vi "RealTimeConversions-CSV.vi"() -> ()   [LabVIEW 2019]
uses:
  <vilib>/userDefined/High Color/IMAQdx.ctl
  <vilib>/vision/driver/NI_Vision_Acquisition_Software.lvlib
  RGB_To_Gray DLL Project/Project RGBToGray VI/RGBToGray.dll
  Gray_To_RGB DLL Project/Gray_to_RGB.dll
panel:
  out "RGB Frame":T1(plugin-control)
  out "GrayScale Frame":T1(plugin-control)
  out "Array":dbl[](array[numeric])
  in  "CSV File Path":path
  out "Elapsed time RGB in sec":dbl
  in  "stop":bool
  out "Camera Frame":T1(plugin-control)
  in  "Available Colormaps":T2
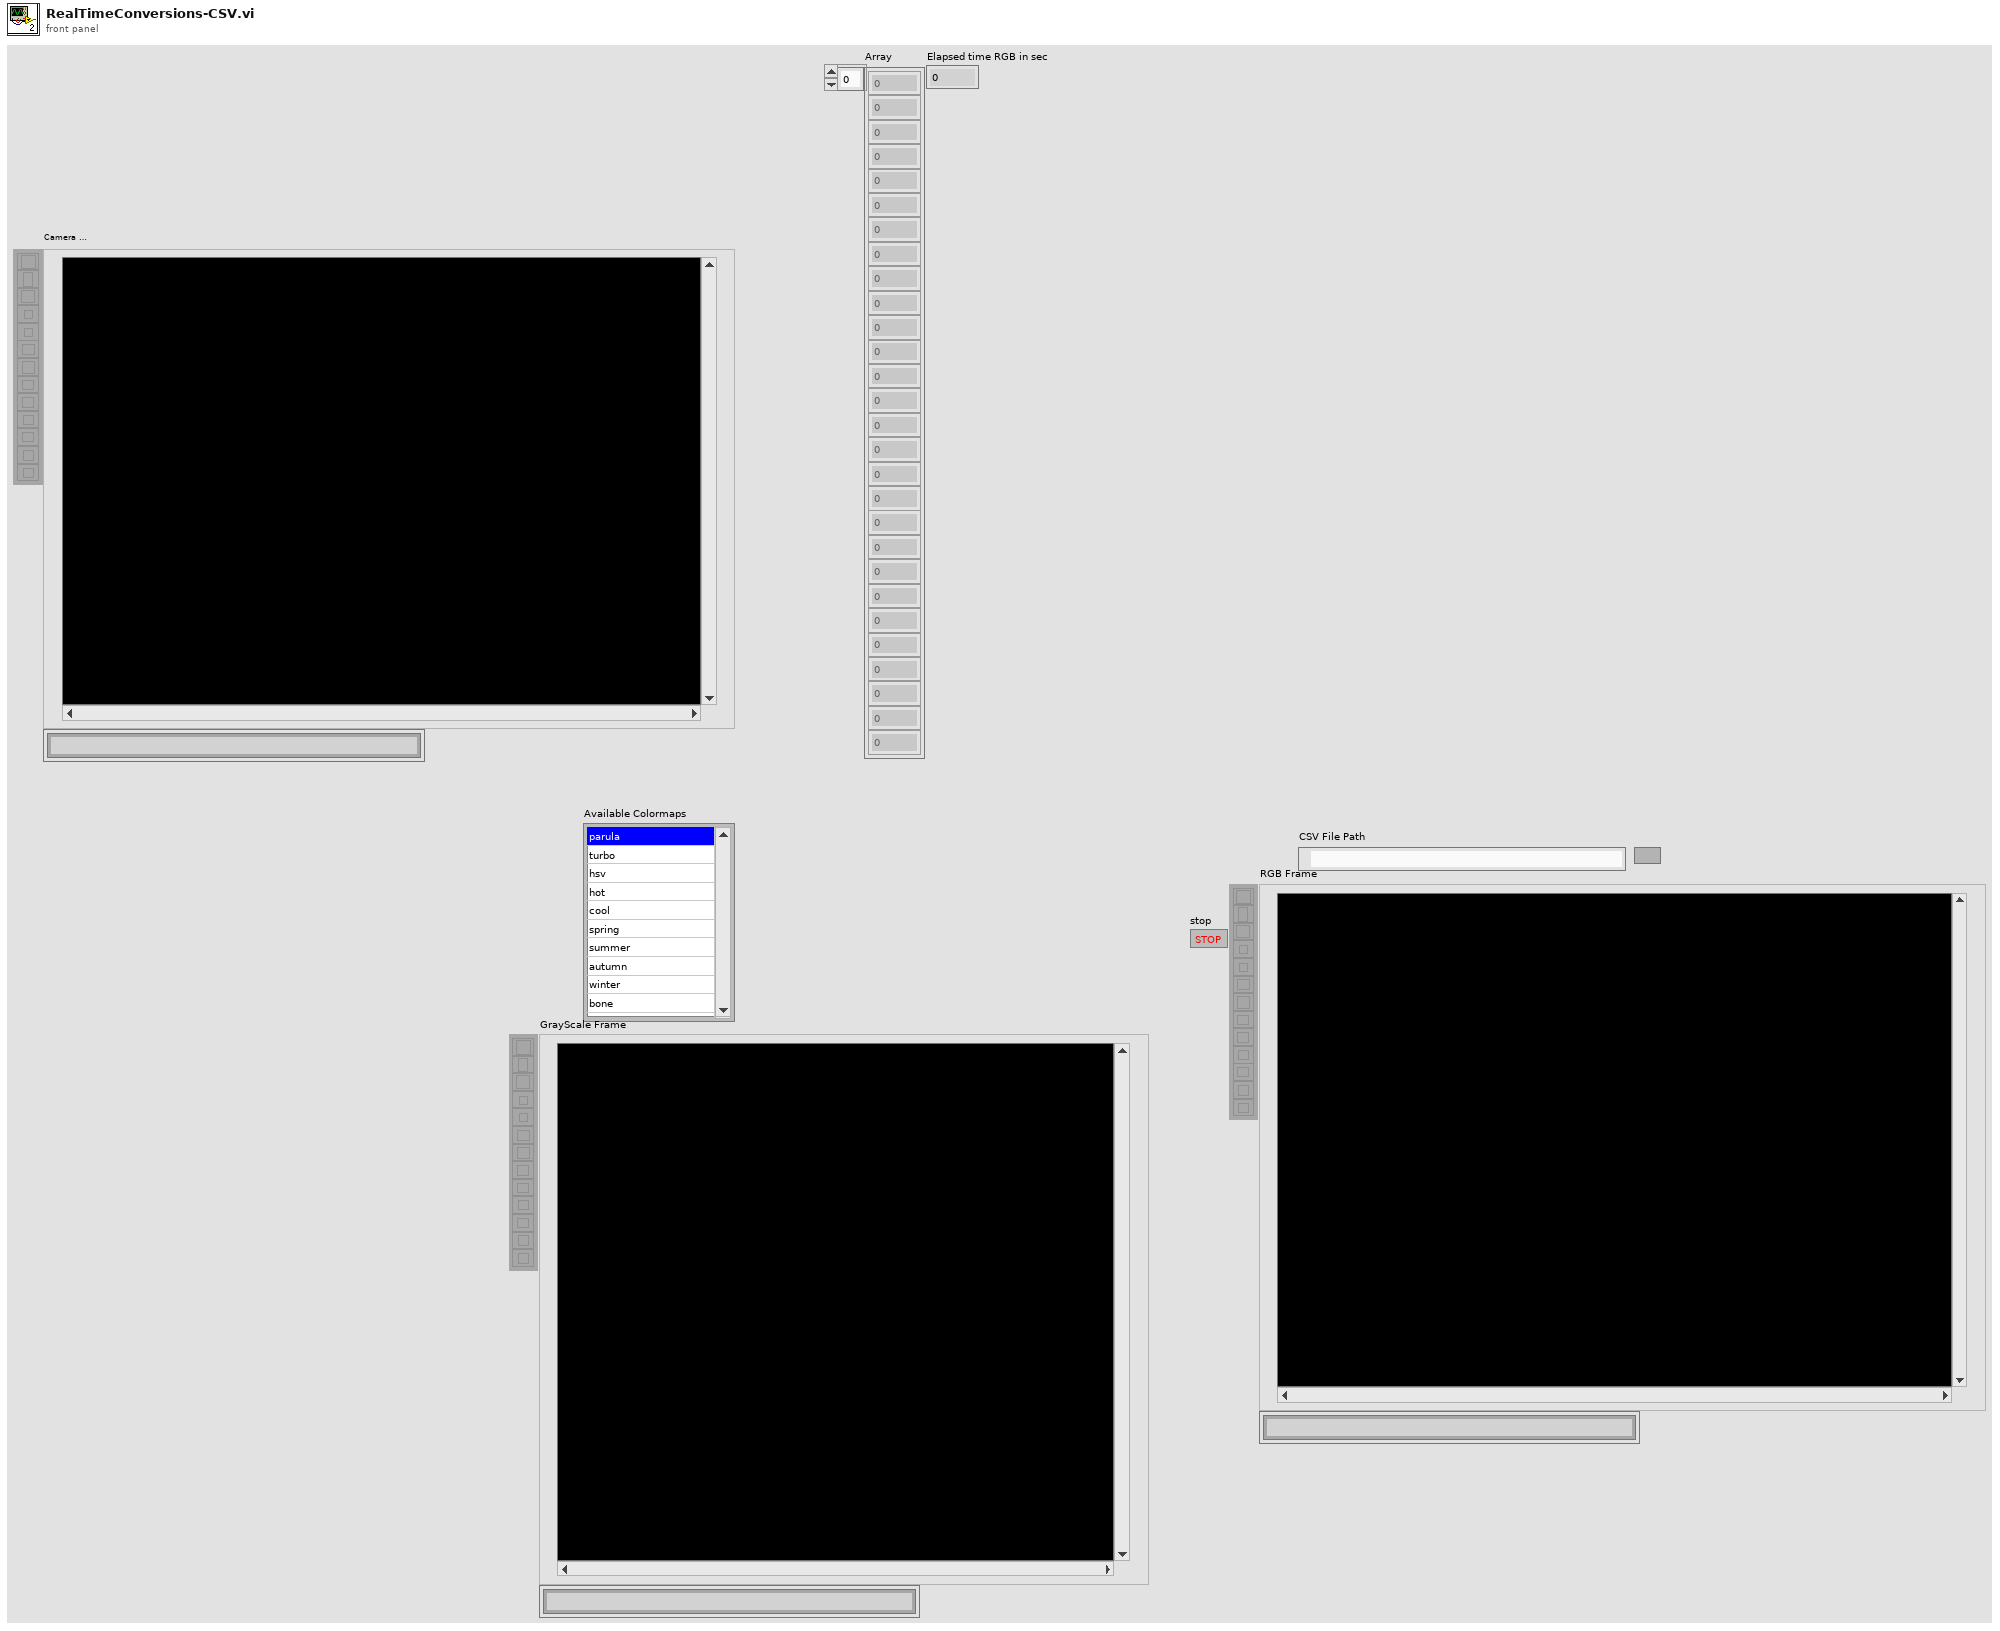
[diagram p1: front panel]
types:
  T1 = typedef "IMAQ Image.ctl" = refnum<image>
  T2 = typedef "Control 1.ctl" = i32
  T3 = typedef "Image Type" = u32
  T4 = typedef "IMAQdx.ctl" = refnum<k21>
  T5 = enum32{"Map Pixel Pointer", "Unmap Pixel Pointer", "Get Pixels Infos"}
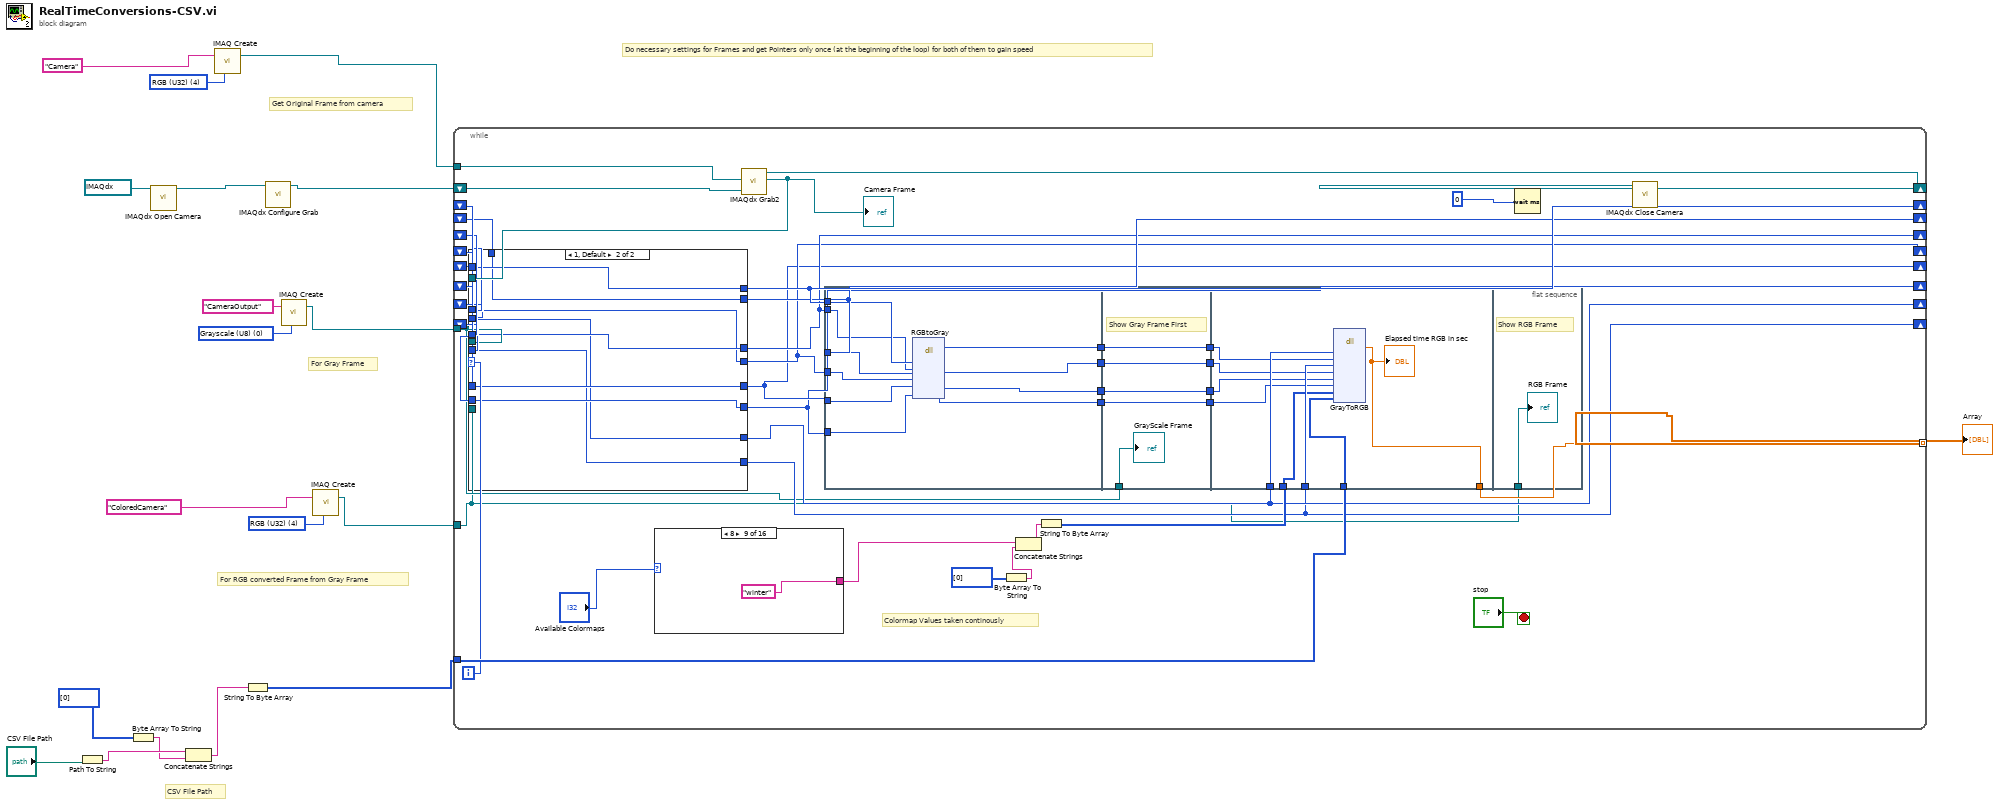
[diagram p0: block diagram]
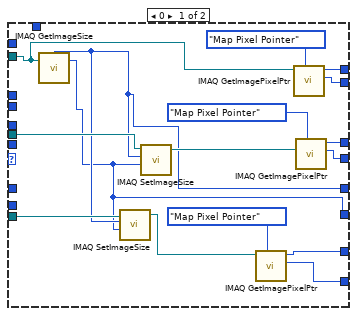
[diagram p2: hidden frame]
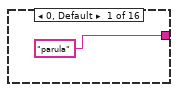
[diagram p3: hidden frame]
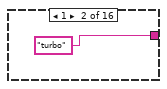
[diagram p4: hidden frame]
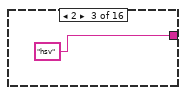
[diagram p5: hidden frame]
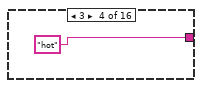
[diagram p6: hidden frame]
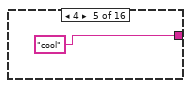
[diagram p7: hidden frame]
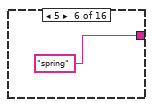
[diagram p8: hidden frame]
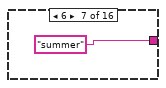
[diagram p9: hidden frame]
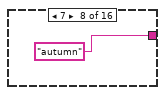
[diagram p10: hidden frame]
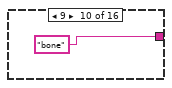
[diagram p11: hidden frame]
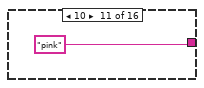
[diagram p12: hidden frame]
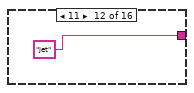
[diagram p13: hidden frame]
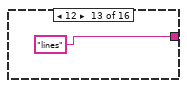
[diagram p14: hidden frame]
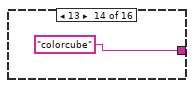
[diagram p15: hidden frame]
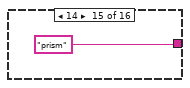
[diagram p16: hidden frame]
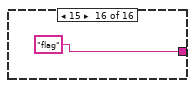
[diagram p17: hidden frame]
diagram:
  w12 = T3 4 items=["Grayscale (U8)", "Grayscale (I16)", "Grayscale (SGL)", "Complex (CSG)", "RGB (U32)", "HSL (U32)", "RGB (U64)", "Grayscale (U16)"] ("Image Type")
  w15 = T3 0 items=["Grayscale (U8)", "Grayscale (I16)", "Grayscale (SGL)", "Complex (CSG)", "RGB (U32)", "HSL (U32)", "RGB (U64)", "Grayscale (U16)"] ("Image Type")
  w17 = T3 4 items=["Grayscale (U8)", "Grayscale (I16)", "Grayscale (SGL)", "Complex (CSG)", "RGB (U32)", "HSL (U32)", "RGB (U64)", "Grayscale (U16)"] ("Image Type")
  # "Do necessary settings for Frames and get Pointers only once (at the beginning of the loop) for both of them to gain speed"
  # "CSV File Path"
  # "For RGB converted Frame from Gray Frame"
  # "For Gray Frame"
  # "Get Original Frame from camera"
  n1 = Path To String(path="CSV File Path") -> (string=w9:string)
  n2 = Byte Array To String(unsigned byte array=u8[] [0]) -> (string=w8:string)
  n3 = call <vilib>:"IMAQdx Open Camera.vi"("Session In"=T4 "cam0") -> ("Session Out"=w19:T4)  [unwired: 9 in, 1 out]
  n4 = Concatenate Strings(w9, w8) -> (w7:string)
  n5 = call "IMAQ Create"("Image Name"="Camera", "Image Type"=w17) -> ("New Image"=w4:T1)  [unwired: 3 in, 1 out]
  n6 = String To Byte Array(string=w7) -> (unsigned byte array=w6:u8[])
  n7 = call <vilib>:"IMAQdx Configure Grab.vi"("Session In"=w19) -> ("Session Out"=w5:T4)  [unwired: 9 in, 1 out]
  n8 = call "IMAQ Create"("Image Name"="CameraOutput", "Image Type"=w15) -> ("New Image"=w2:T1)  [unwired: 3 in, 1 out]
  n9 = call "IMAQ Create"("Image Name"="ColoredCamera", "Image Type"=w12) -> ("New Image"=w3:T1)  [unwired: 3 in, 1 out]
  n10 = while {
    shift-right: [w59] -> w14
    shift-left: w5 -> [w61]
    tunnel: w6 -> [w57]
    tunnel: w3 -> [w21]
    tunnel: w4 -> [w50]
    tunnel: w2 -> [w23]
    shift-right: [w47] -> _
    shift-left: _ -> [w45]
    shift-right: [w46] -> _
    shift-left: _ -> [w44]
    shift-right: [w43] -> _
    shift-left: _ -> [w42]
    shift-right: [w41] -> _
    shift-left: _ -> [w40]
    shift-right: [w39] -> _
    shift-left: _ -> [w38]
    shift-right: [w37] -> _
    shift-left: _ -> [w36]
    shift-right: [w35] -> _
    shift-left: _ -> [w34]
    shift-right: [w33] -> _
    shift-left: _ -> [w32]
    tunnel: [w22] -> w1 mode=indexing
    i -> [w49]
    stop <- "stop" stop-if-true
    # "Colormap Values taken continously"
    n11 = case shown="8" "Available Colormaps" {
      tunnel: ["parula" "turbo" "hsv" "hot" "cool" "spring" "summer" "autumn" "winter" "bone" "pink" "jet" "lines" "colorcube" "prism" "flag"] -> w52
      frame 0, Default {
      }
      frame 1 {
      }
      frame 2 {
      }
      frame 3 {
      }
      frame 4 {
      }
      frame 5 {
      }
      frame 6 {
      }
      frame 7 {
      }
      frame 8 {
      }
      frame 9 {
      }
      frame 10 {
      }
      frame 11 {
      }
      frame 12 {
      }
      frame 13 {
      }
      frame 14 {
      }
      frame 15 {
      }
    }
    n12 = call <vilib>:"IMAQdx Grab2.vi"("Image In"=w50, "Session In"=w61) -> ("Image Out"=w48:T1, "Session Out"=w59:T4)  [unwired: 6 in, 2 out]
    "Camera Frame" <- w48
    n13 = case shown="1, Default" w49 {
      tunnel: w48 -> [w66 _]
      tunnel: w23 -> [w72 _]
      tunnel: w21 -> [w71 _]
      tunnel: [w70 w79] -> w35
      tunnel: [w69 w78] -> w33
      tunnel: [w68 w83] -> w43
      tunnel: [w67 w82] -> w41
      tunnel: [w65 w81] -> w39
      tunnel: [w64 w80] -> w37
      tunnel: [w63 w85] -> w47
      tunnel: [w62 w84] -> w46
      tunnel: w45 -> [_ w85]
      tunnel: w44 -> [_ w84]
      tunnel: w42 -> [_ w83]
      tunnel: w40 -> [_ w82]
      tunnel: w38 -> [_ w81]
      tunnel: w36 -> [_ w80]
      tunnel: w34 -> [_ w79]
      tunnel: w32 -> [_ w78]
      frame 0 {
        n14 = call "IMAQ GetImageSize"("Image"=w66) -> ("Y Resolution"=w64:i32, "X Resolution"=w65:i32)  [unwired: 3 in, 1 out]
        n15 = call "IMAQ SetImageSize"("Y Resolution"=w64, "X Resolution"=w65, "Image"=w71) -> ("Image Out"=w75:T1)  [unwired: 2 in, 1 out]
        n16 = call "IMAQ SetImageSize"("Y Resolution"=w64, "X Resolution"=w65, "Image"=w72) -> ("Image Out"=w73:T1)  [unwired: 2 in, 1 out]
        n17 = call "IMAQ GetImagePixelPtr"("Function"=T5."Map Pixel Pointer", "Image"=w75) -> ("LineWidth(Pixels)"=w69:i32, "Pixel Pointer out"=w70:u64)  [unwired: 4 in, 4 out]
        n18 = call "IMAQ GetImagePixelPtr"("Function"=T5."Map Pixel Pointer", "Image"=w66) -> ("LineWidth(Pixels)"=w62:i32, "Pixel Pointer out"=w63:u64)  [unwired: 4 in, 4 out]
        n19 = call "IMAQ GetImagePixelPtr"("Function"=T5."Map Pixel Pointer", "Image"=w73) -> ("LineWidth(Pixels)"=w67:i32, "Pixel Pointer out"=w68:u64)  [unwired: 4 in, 4 out]
      }
      frame 1, Default {
      }
    }
    n20 = flat-sequence {
      tunnel: [w111] -> w31
      tunnel: [w110] -> w29
      tunnel: [w109] -> w27
      tunnel: [w108] -> w25
      tunnel: w47 -> [w107]
      tunnel: w43 -> [w106]
      tunnel: w46 -> [w105]
      tunnel: w41 -> [w104]
      tunnel: w39 -> [w103]
      tunnel: w37 -> [w102]
      tunnel: w31 -> [w116]
      tunnel: [w116] -> w30
      tunnel: w29 -> [w115]
      tunnel: [w115] -> w28
      tunnel: w27 -> [w114]
      tunnel: [w114] -> w26
      tunnel: w25 -> [w113]
      tunnel: [w113] -> w24
      tunnel: w23 -> [w112]
      tunnel: w51 -> [w119]
      tunnel: w57 -> [w118]
      tunnel: w30 -> [w124]
      tunnel: w28 -> [w122]
      tunnel: w26 -> [w121]
      tunnel: w24 -> [w120]
      tunnel: w35 -> [w125]
      tunnel: w33 -> [w123]
      tunnel: [w117] -> w22
      tunnel: w21 -> [w126]
      frame #0 {
        n21 = dll-call lib="C:/Users/byald/Desktop/EE-433 Project Group1/RGB_To_Gray DLL Project/Project RGBToGray VI/RGBToGray.dll" fn="RGBtoGray"("RGBImage"=w107, "GrayImage"=w106, "LVLineWidthRGB"=w105, "LVLineWidthGray"=w104, "LVWidth"=w103, "LVHeight"=w102) -> ("GrayImage"=w111:u64, "LVLineWidthGray"=w110:i32, "LVWidth"=w109:i32, "LVHeight"=w108:i32)  [unwired: 6 in, 2 out]
      }
      frame #1 {
        # "Show Gray Frame First"
        "GrayScale Frame" <- w112
      }
      frame #2 {
        n22 = dll-call lib="C:/Users/byald/Desktop/EE-433 Project Group1/Gray_To_RGB DLL Project/Gray_to_RGB.dll" fn="GrayToRGB"("RGBImage"=w125, "GrayImage"=w124, "LVLineWidthRGB"=w123, "LVLineWidthGray"=w122, "LVWidth"=w121, "LVHeight"=w120, "ColorMap"=w119, "CsvPath"=w118) -> ("return type"=w117:dbl)  [unwired: 11 in, 2 out]
        "Elapsed time RGB in sec" <- w117
      }
      frame #3 {
        # "Show RGB Frame"
        "RGB Frame" <- w126
      }
    }
    n23 = Byte Array To String(unsigned byte array=u8[] [0]) -> (string=w54:string)
    n24 = Concatenate Strings(w52, w54) -> (w53:string)
    n25 = String To Byte Array(string=w53) -> (unsigned byte array=w51:u8[])
    n26 = Wait (ms)(milliseconds to wait=u32 0) -> ()  [unwired: 1 out]
  }
  "Array" <- w1
  n27 = call <vilib>:"IMAQdx Close Camera.vi"("Session In"=w14) -> ()  [unwired: 10 in, 1 out]
